vi "Overview Draw Bounding.vi"(8 "error in (no error)":errorcluster, 10 "Color":u32(colorbox), 11 "XYGraphOverview in":refnum<class "XYGraphOverview.lvclass">) -> (0 "error out":errorcluster, 3 "XYGraphOverview out":refnum<class "XYGraphOverview.lvclass">)   [LabVIEW 2020, in "XYGraphOverview.lvlib" / "XYGraphOverview.lvclass"]
uses:
  XYGraphOverview.lvclass
  XYGraphOverview.lvclass/XYGraphOverview.ctl
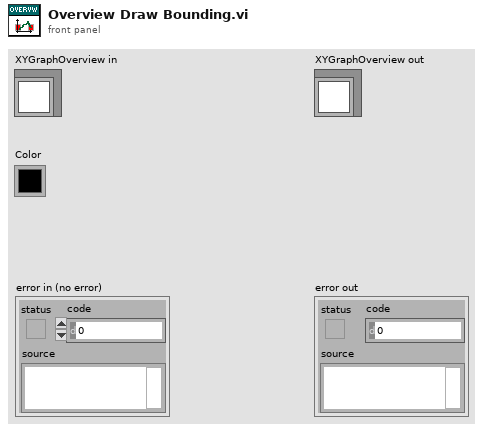
[diagram p1: front panel]
types:
  T1 = cluster{"left":i16, "top":i16, "right":i16, "bottom":i16}
  T2 = typedef "LVRectTypeDef.ctl" = cluster{"Left":i16, "Top":i16, "Right":i16, "Bottom":i16}
  T3 = typedef "LVPoint32TypeDef.ctl" = cluster{"Horizontal":i32, "Vertical":i32}
  T4 = cluster{"Left":i32, "Top":i32, "Right":i32, "Bottom":i32}
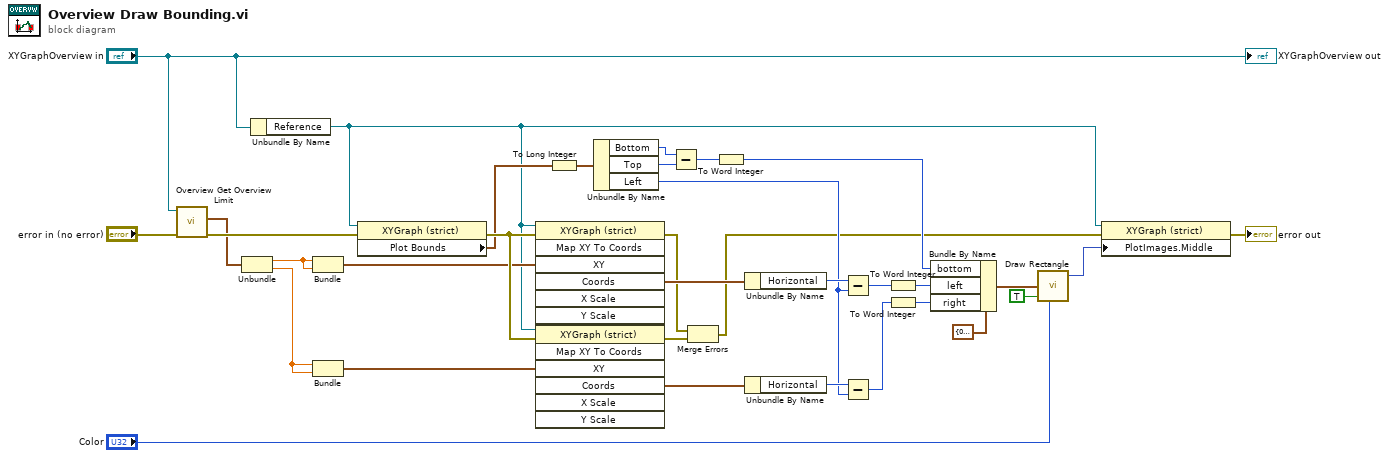
[diagram p0: block diagram]
diagram:
  n1 = call "Overview Get Overview Limit.vi"("error in"="error in (no error)", "XYGraphOverview in"="XYGraphOverview in") -> ("error out"=w7:errorcluster, "Limit"=w4:cluster{"Lower Limit":dbl, "Upper Limit":dbl})  [unwired: 7 in, 1 out]
  n2 = Unbundle(w4) -> ("Lower Limit"=w6:dbl, "Upper Limit"=w5:dbl)
  n3 = Unbundle By Name("XYGraphOverview in") -> ("Reference"=w3:refnum<vi>)
  n4 = Bundle("Lower Limit"=w6, "Lower Limit"=w6) -> (w11:cluster{"Lower Limit":dbl, "Lower Limit":dbl})  [unwired: 1 in]
  n5 = Bundle("Upper Limit"=w5, "Upper Limit"=w5) -> (w10:cluster{"Upper Limit":dbl, "Upper Limit":dbl})  [unwired: 1 in]
  n6 = property on="Property Node" class="XYGraph (strict)"(reference=w3, error in=w7) -> (error out=w34:errorcluster, "Plot Bounds"=w30:T2)  [unwired: 1 out]
  n7 = invoke on="Invoke Node" class="XYGraph (strict)" method="Map XY To Coords"(reference=w3, error in=w34, "XY"=w11) -> (error out=w19:errorcluster, "Coords"=w33:T3)  [unwired: 4 in, 5 out]
  n8 = invoke on="Invoke Node" class="XYGraph (strict)" method="Map XY To Coords"(reference=w3, error in=w34, "XY"=w10) -> (error out=w20:errorcluster, "Coords"=w32:T3)  [unwired: 4 in, 5 out]
  n9 = To Long Integer(number=w30) -> (32bit integer=w31:T4)
  n10 = Unbundle By Name(w31) -> ("Bottom"=w17:i32, "Top"=w18:i32, "Left"=w14:i32)
  n11 = Subtract(x=w17, y=w18) -> (x-y=w16:i32)
  n12 = Merge Errors(w19, w20) -> (w2:errorcluster)
  n13 = To Word Integer(number=w16) -> (16bit integer=w15:i16)
  n14 = Unbundle By Name(w33) -> ("Horizontal"=w29:i32)
  n15 = Unbundle By Name(w32) -> ("Horizontal"=w28:i32)
  n16 = Subtract(x=w29, y=w14) -> (x-y=w22:i32)
  n17 = Subtract(x=w28, y=w14) -> (x-y=w21:i32)
  n18 = To Word Integer(number=w22) -> (16bit integer=w26:i16)
  n19 = To Word Integer(number=w21) -> (16bit integer=w27:i16)
  n20 = Bundle By Name(cluster=T1 {"left"=0, "top"=0, "right"=0, "bottom"=500} ("rect"), "bottom"=w15, "left"=w26, "right"=w27) -> (w24:T1)
  n21 = call <vilib>:"Draw Rectangle.vi"("rect"=w24, "fill?(F)"=TRUE, "color(black)"="Color") -> ("new picture"=w13:picture)  [unwired: 6 in]
  n22 = property on="Property Node" class="XYGraph (strict)"(reference=w3, error in=w2, "PlotImages.Middle"=w13) -> (error out=→"error out":errorcluster)  [unwired: 1 out]
  "XYGraphOverview out" <- "XYGraphOverview in"
